vi "Write Byte.vi"(8 "error in (no error)":errorcluster, 9 "Value":u8 format="%.0b", 10 "Reg Address":T3, 11 "Chip Address (A2 A1 A0)":T2 max=7) -> (0 "error out":errorcluster, 3 "SPI Command":T1)   [LabVIEW 2014, in "SLSC configuration Shared.lvlib"]
doc: "Writes a byte of data to a desired register address."
uses:
  IOCON BANK 0 Reg Addresses.ctl
  Chip Address.ctl
  SPI Command.ctl
  OPCODE.ctl
  CD/Source/Shared/SLSC configuration Shared.lvlib
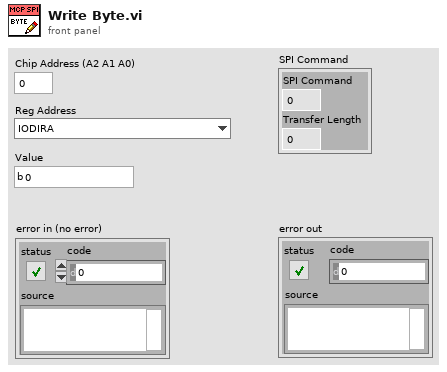
[diagram p1: front panel]
types:
  T1 = typedef "SLSC configuration Shared.lvlib/SPI Command.ctl" = cluster{"SPI Command":u32, "Transfer Length":u8}
  T2 = typedef "SLSC configuration Shared.lvlib/Chip Address.ctl" = u8
  T3 = typedef "SLSC configuration Shared.lvlib/IOCON BANK 0 Reg Addresses.ctl" = enum8{"IODIRA", "IODIRB", "IPOLA", "IPOLB", "GPINTENA", "GPINTENB", "DEFVALA", "DEFVALB", "INTCONA", "INTCONB", "IOCONA", "IOCONB", "GPPUA", "GPPUB", "INTFA", "INTFB", "INTCAPA", "INTCAPB", "GPIOA", "GPIOB", "OLATA", "OLATB"}
  T4 = typedef "SLSC configuration Shared.lvlib/OPCODE.ctl" = u8
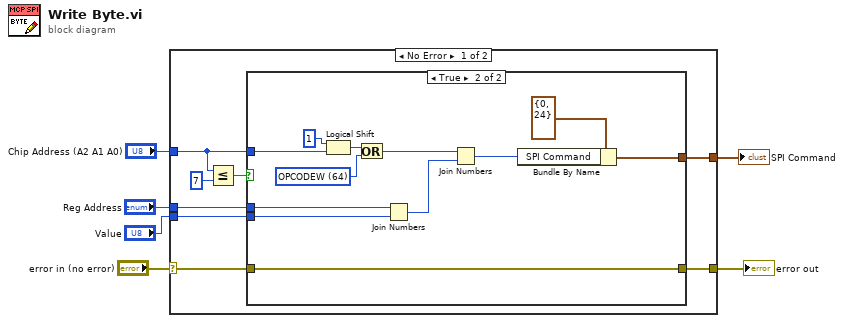
[diagram p0: block diagram]
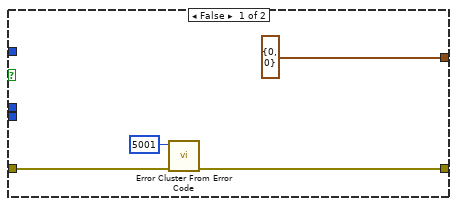
[diagram p2: hidden frame]
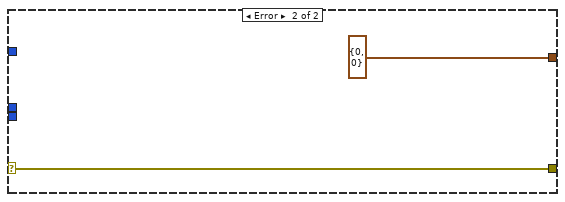
[diagram p3: hidden frame]
diagram:
  n1 = case shown="No Error" "error in (no error)" {
    selector: "error in (no error)" -> [w8 w32]
    tunnel: "Reg Address" -> [w14 _]
    tunnel: "Value" -> [w13 _]
    tunnel: "Chip Address (A2 A1 A0)" -> [w11 _]
    tunnel: [w9 w32] -> w3
    tunnel: [w7 T1 {"SPI Command"=0, "Transfer Length"=0} ("SPI Command 2")] -> w1
    frame No Error {
      n2 = Less Or Equal?(x=w11, y=T2 7) -> (x <= y?=w10:bool)
      n3 = case shown="True" w10 {
        tunnel: w11 -> [_ w27]
        tunnel: w14 -> [_ w26]
        tunnel: w13 -> [_ w25]
        tunnel: [w17 w22] -> w9
        tunnel: w8 -> [w16 w22]
        tunnel: [T1 {"SPI Command"=0, "Transfer Length"=0} ("SPI Command 2") w19] -> w7
        frame False {
          n4 = call <vilib>:"Error Cluster From Error Code.vi"("error in (no error)"=w16, "error code (0)"=5001) -> ("error out"=w17:errorcluster)  [unwired: 7 in]
        }
        frame True {
          w28 = T4 64 items=["OPCODEW"=64, "OPCODER"=65] ("OPCODE")
          n5 = Logical Shift(y=i16 1, x=w27) -> (x << y=w29:T2)
          n6 = Or(x=w29, y=w28) -> (x .or. y?=w23:T2)
          n7 = Join Numbers(hi=w26, lo=w25) -> ((hi.lo)=w24:u16)
          n8 = Join Numbers(hi=w23, lo=w24) -> ((hi.lo)=w20:u32)
          n9 = Bundle By Name(cluster=T1 {"SPI Command"=0, "Transfer Length"=24} ("SPI Command 2"), "SPI Command"=w20) -> (w19:T1)
        }
      }
    }
    frame Error {
    }
  }
  "error out" <- w3
  "SPI Command" <- w1
